vi "Dresser DXD Read Heise Label.vi"(0 "VISA session":refnum<visa-resource-name>, 5 "DXD Address (1)":T1=1 min=1 max=99 step=1, 11 "Error In (no error)":errorcluster) -> (4 "dup VISA session":refnum<visa-resource-name>, 6 "Returned String":string, 8 "Heise Label (S/N)":string="000000", 15 "Error Out":errorcluster)   [LabVIEW 2015]
doc: "This VI will read the Heise label (serial number) from the Dresser DXD Series pressure transducer. This number should correspond to the number printed on the transducer label.\n\nWritten by:\nBLOOMY CONTROLS, INC\nWINDSOR, CT 06095, USA\n860-298-9925\nwww.bloomy.com\nV2.0.0\nMay, 2002"
uses:
  Type Defs/DXD Address.ctl
panel:
  # "For instructions on the use of this VI, press Ctrl+H to display the help window and move the mouse over the icon, controls, and indicators"
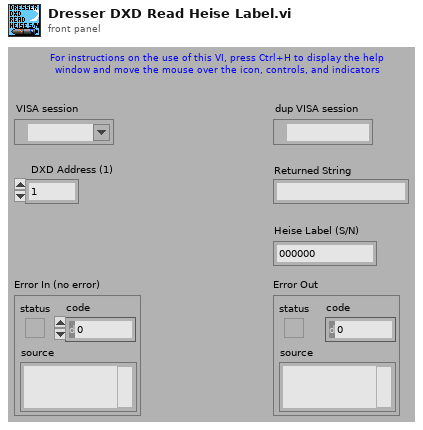
[diagram p1: front panel]
types:
  T1 = typedef "DXD Address.ctl" = i32
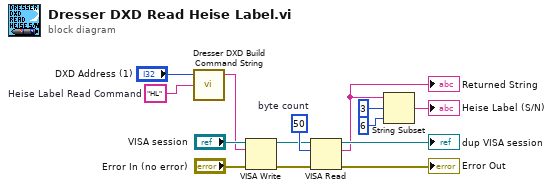
[diagram p0: block diagram]
diagram:
  w9 = u32 50  # byte count
  w10 = "HL"  # Heise Label Read Command
  n1 = call "Dresser DXD Build Command String.vi"("Command Mnemonic (\"\")"=w10, "DXD Address (1)"="DXD Address (1)") -> ("Command String"=w12:string)  [unwired: 3 in]
  n2 = VISA Write(VISA resource name="VISA session", write buffer=w12, error in (no error)="Error In (no error)") -> (VISA resource name out=w8:refnum<visa-resource-name>, error out=w7:errorcluster)  [unwired: 1 out]
  n3 = VISA Read(VISA resource name=w8, byte count=w9, error in (no error)=w7) -> (VISA resource name out=→"dup VISA session":refnum<visa-resource-name>, read buffer=w2:string, error out=→"Error Out":errorcluster)  [unwired: 1 out]
  "Returned String" <- w2
  n4 = String Subset(string=w2, offset (0)=3, length (rest)=6 ("length (rest)")) -> (substring=→"Heise Label (S/N)":string)
